vi "Relink CFG Files to new Directory.vi"() -> ()   [LabVIEW 2020]
uses:
  <vilib>/Utility/config.llb/Read Key (Path).vi
  <vilib>/Utility/config.llb/Write Key (Path).vi
  <vilib>/Utility/config.llb/NI_LVConfig.lvlib
panel:
  out "error out":errorcluster
  in  "Destination Folder":path=path "C:/Program Files/Westinghouse/IVMS_SG/Configuration"
  in  "section":string="DAQmxConfigurationFiles"
  in  "error in (no error)":errorcluster
  in  "configuration file path":path=path "C:/Program Files/Westinghouse/IVMS_SG/Configuration/DAQmx_TaskList.cfg"
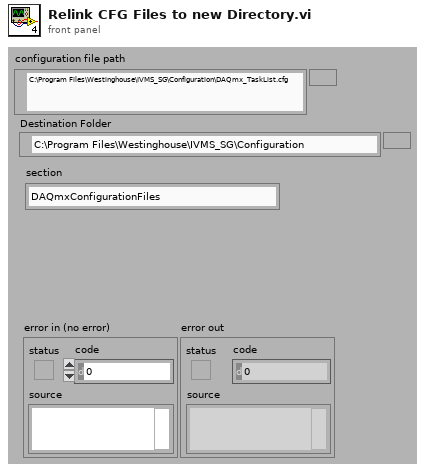
[diagram p1: front panel]
types:
  T1 = typedef "NI_LVConfig.lvlib/Config Data RefNum.ctl" = refnum<k1>
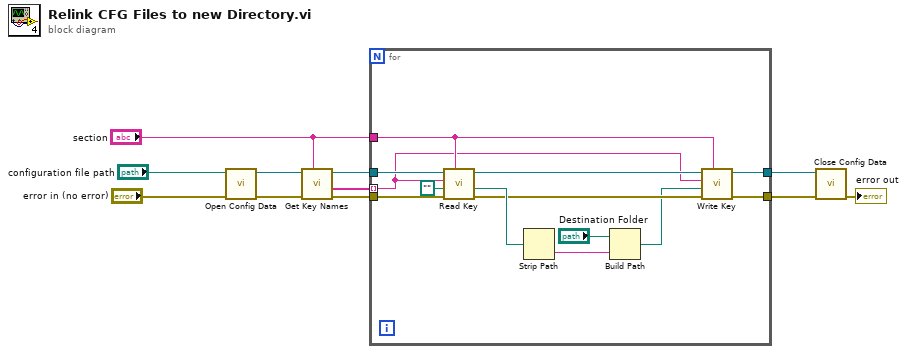
[diagram p0: block diagram]
diagram:
  n1 = call <vilib>:"Open Config Data.vi"("error in (no error)"="error in (no error)", "configuration file path"="configuration file path") -> ("error out"=w11:errorcluster, "refnum"=w10:T1)  [unwired: 7 in, 1 out]
  n2 = call <vilib>:"Get Key Names.vi"("section"="section", "error in (no error)"=w11, "refnum"=w10) -> ("error out"=w7:errorcluster, "key names"=w4:string[], "refnum out"=w6:T1)  [unwired: 5 in, 1 out]
  n3 = for {
    tunnel: w7 -> [w24]
    tunnel: w6 -> [w22]
    tunnel: "section" -> [w17]
    tunnel: w4 -> [w15] mode=indexing
    tunnel: [w13] -> w3
    tunnel: [w12] -> w2
    n4 = call-poly <vilib>:"Read Key.vi"("section"=w17, "error in (no error)"=w24, "default value"=path "", "key"=w15, "refnum"=w22) -> ("error out"=w16:errorcluster, "value"=w21:path, "refnum out"=w18:T1)  [unwired: 3 in, 1 out]
    n5 = Strip Path(path=w21) -> (name=w20:string)  [unwired: 1 out]
    n6 = Build Path(base path="Destination Folder", name or relative path=w20) -> (appended path=w14:path)
    n7 = call-poly <vilib>:"Write Key.vi"("section"=w17, "error in (no error)"=w16, "value"=w14, "key"=w15, "refnum"=w18) -> ("error out"=w13:errorcluster, "refnum out"=w12:T1)  [unwired: 4 in, 1 out]
  }
  n8 = call <vilib>:"Close Config Data.vi"("error in (no error)"=w3, "refnum"=w2) -> ("error out"=→"error out":errorcluster)  [unwired: 8 in, 1 out]
